vi "Rotate.vi"   [LabVIEW 2020, in "image.lvlib"]
uses:
  image.lvlib
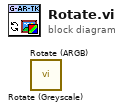
[diagram p0: block diagram]
diagram:
  n1 = call "Rotate (Greyscale).vi"() -> ()  [unwired: 10 in, 2 out]
  n2 = call "Rotate (ARGB).vi"() -> ()  [unwired: 10 in, 2 out]
